vi "TDMS - File Viewer (NXG Style).vi"(8 "error in":errorcluster, 11 "file in":path) -> (0 "error out":errorcluster={"status"=TRUE, "code"=118, "source"="TDMS Open in TDMS - File Viewer with Flat Layout.vi"}, 3 "file out":path)   [LabVIEW 2020, in "NI_TDMS File Viewer.lvlib"]
doc: "Opens the .tdms file specified in the <B>file path</B> input and presents the file data in the TDMS File Viewer dialog box."
uses:
  <vilib>/Utility/TDMS File Viewer/NI_TDMS File Viewer.lvlib
  <vilib>/Utility/miscctls.llb/LVRowAndColumnTypeDef.ctl
  <vilib>/Utility/error.llb/DialogType.ctl
  <vilib>/Utility/TDMS File Viewer/Global VI for Localized Text.vi
panel:
  in  "Help":bool
  in  "File Tree":string[](tree)
  out "Property Table":string[][](table)
  in  "All":bool
  in  "Samples":i64=100000 min=-1 step=1
  in  "Start index":i64 min=0 step=1
  out "Waveform Graph":waveform(dbl)[](graph)
  in  "Value Table":i32(listbox)=-1
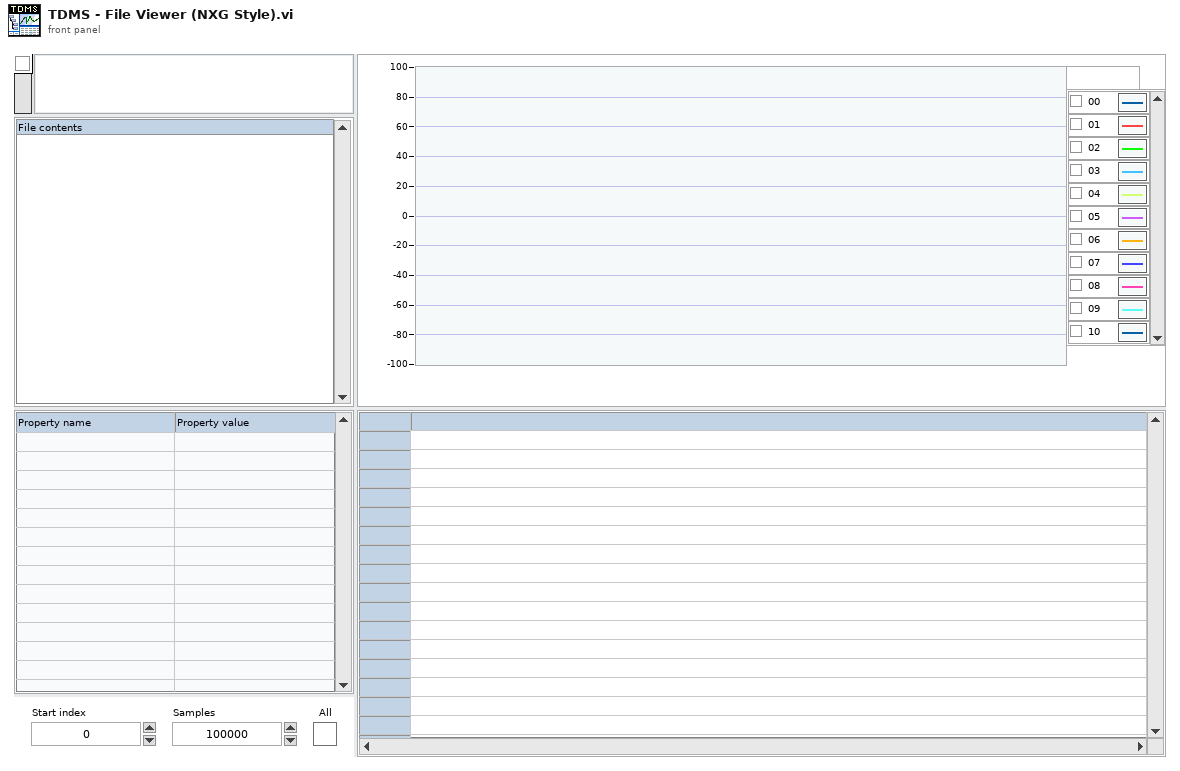
[diagram p1: front panel]
types:
  T1 = enum16{"open", "open or create", "create or replace", "create", "open (read-only)"}
  T2 = cluster{"All":bool, "Start index":i64, "Samples":i64}
  T3 = enum8{"Enabled", "Disabled", "Disabled and Grayed Out"}
  T4 = typedef "eventvkey.ctl" = enum16{"ASCII", "Enter", "Return", "Shift", "Ctrl", "Alt", "Cmd", "Opt", "Caps", "NumLock", "Clear", "Break", "Up", "Down", "Left", "Right", "Insert", "Delete", "Home", "End", "PageUp", "PageDown", "Escape", "Help", "Pause", "ScrollLock", "F1", "F2", "F3", "F4", "F5", "F6", "F7", "F8", "F9", "F10", "F11", "F12", "F13", "F14", "F15", "F16", "F17", "F18", "F19", "F20", "F21", "F22", "F23", "F24", "Play", "VolumeUp", "VolumeDown", "Mute", "Two Byte Char"}
  T5 = typedef "LVPoint32TypeDef.ctl" = cluster{"Horizontal":i32, "Vertical":i32}
  T6 = typedef "NI_TDMS File Viewer.lvlib/Table Components.ctl" = cluster{"column headers":string[], "row headers":string[], "values":string[][]}
  T7 = typedef "LVRowAndColumnTypeDef.ctl" = cluster{"Row":i32, "Column":i32}
  T8 = typedef "DialogType.ctl" = u16
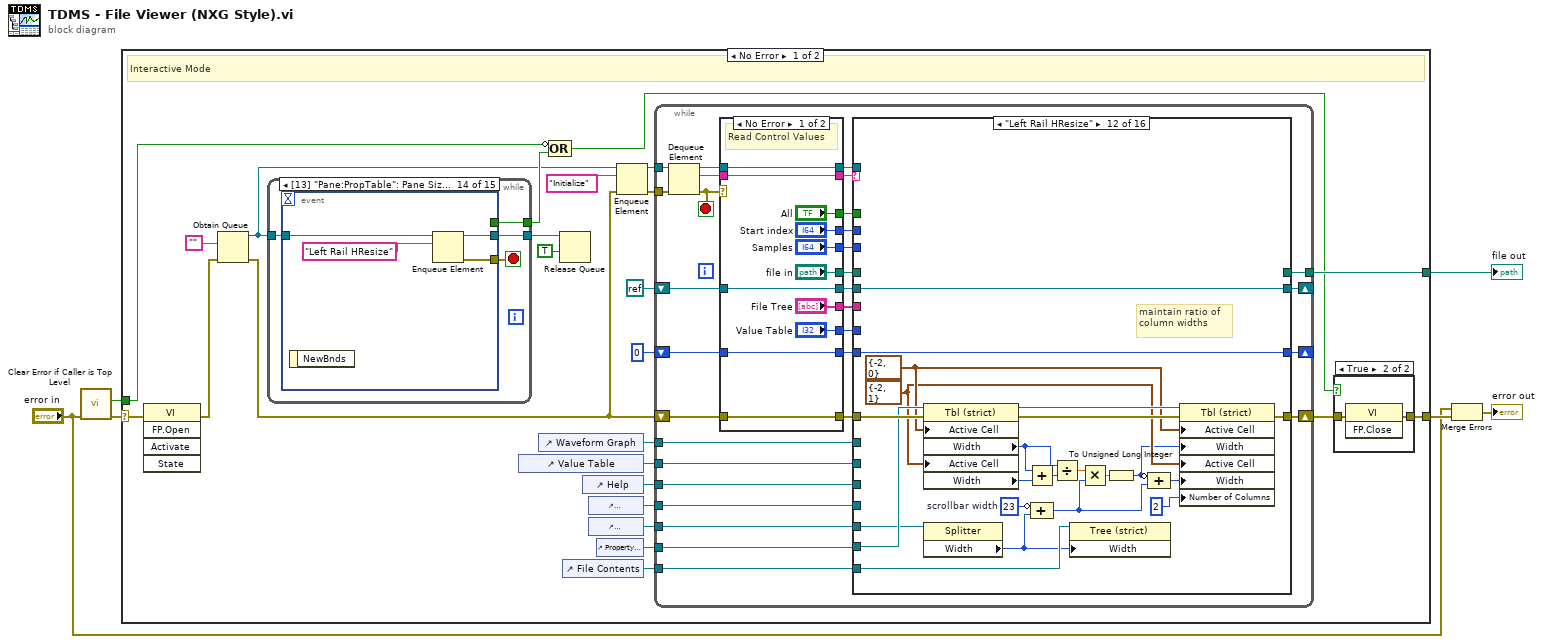
[diagram p0: block diagram]
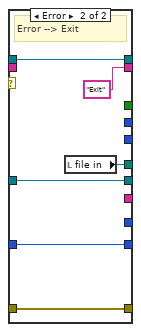
[diagram p3: hidden frame]
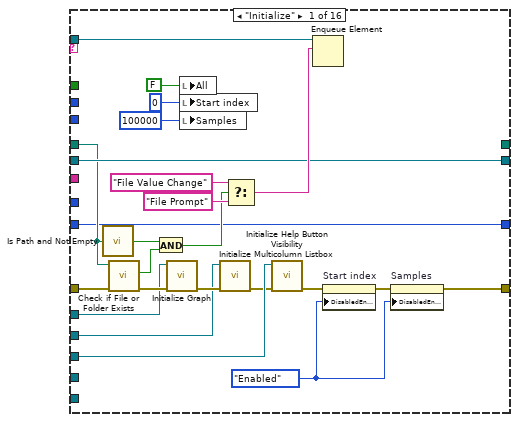
[diagram p4: hidden frame]
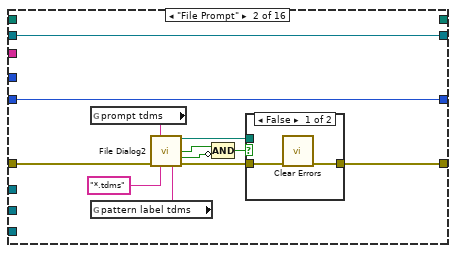
[diagram p5: hidden frame]
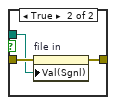
[diagram p6: hidden frame]
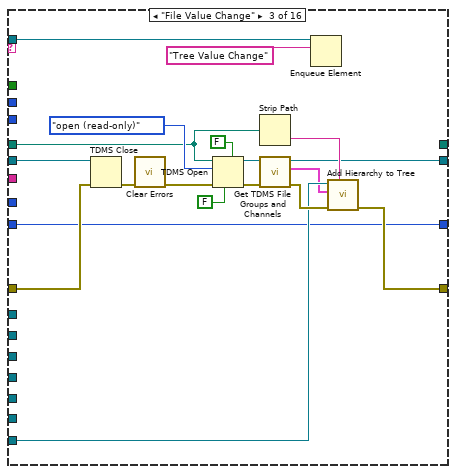
[diagram p7: hidden frame]
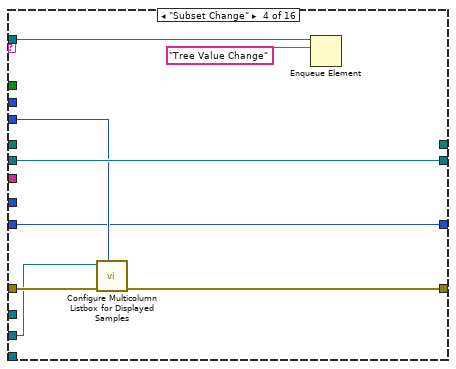
[diagram p8: hidden frame]
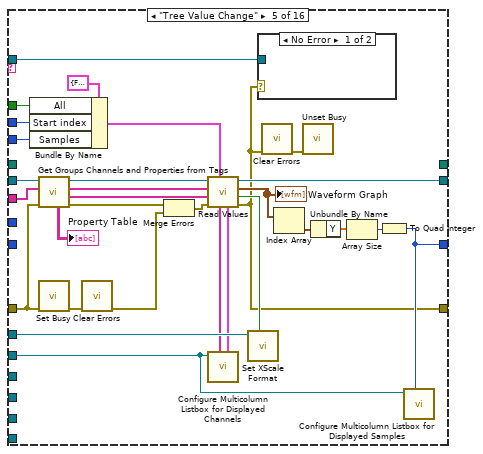
[diagram p9: hidden frame]
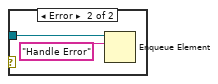
[diagram p10: hidden frame]
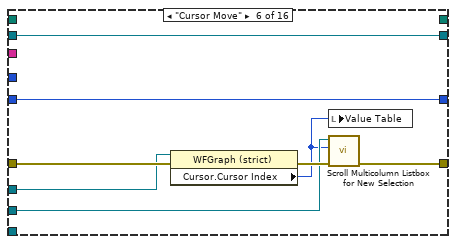
[diagram p11: hidden frame]
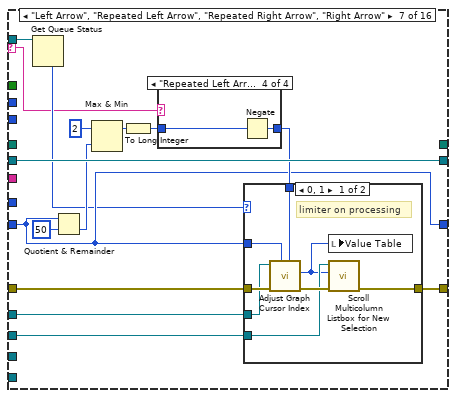
[diagram p12: hidden frame]
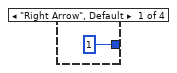
[diagram p14: hidden frame]
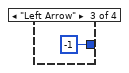
[diagram p16: hidden frame]
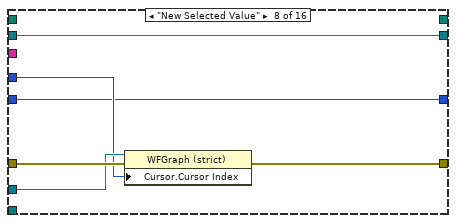
[diagram p17: hidden frame]
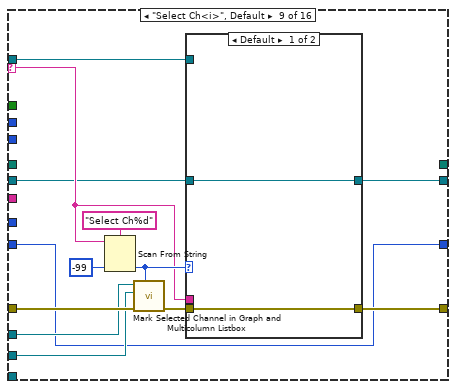
[diagram p18: hidden frame]
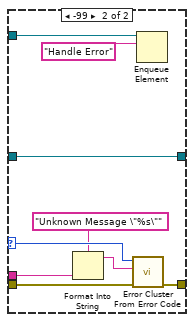
[diagram p19: hidden frame]
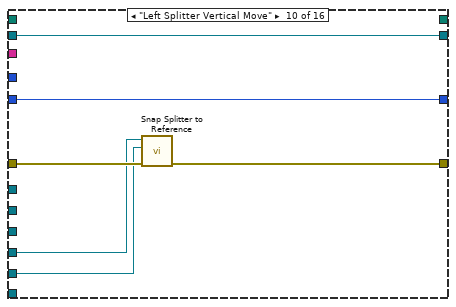
[diagram p20: hidden frame]
diagram:
  n1 = call <vilib>:"Clear Error if Caller is Top Level.vi"("error in"="error in") -> ("error out"=w6:errorcluster, "top level"=w1:bool)  [unwired: 9 in]
  n2 = case shown="No Error" w6 {
    selector: w6 -> [w11 w429]
    tunnel: [w21 _] -> w2
    tunnel: [w30 w429] -> w5
    tunnel: w1 -> [w18 _]
    frame No Error {
      # "Interactive Mode"
      n3 = invoke class="VI" method="FP.Open"(error in=w11) -> (error out=w10:errorcluster)  [unwired: 4 in, 4 out]
      n4 = Obtain Queue(element data type="", error in (no error)=w10) -> (queue out=w9:refnum<queue>, error out=w12:errorcluster)  [unwired: 3 in, 1 out]
      n5 = while {
        tunnel: [w315] -> w20
        tunnel: w9 -> [w314]
        tunnel: [w313] -> w16
        stop <- w316 stop-if-true
        n6 = event shown="[13] \"Pane:PropTable\": Pane Size" {
          selector: _ -> [_ _ _ _ _ _ _ _ _ _ _ _ _ _ _]
          dyn-events: _ -> [_ _ _ _ _ _ _ _ _ _ _ _ _ _ _]
          timeout: _ -> [_ _ _ _ _ _ _ _ _ _ _ _ _ _ _]
          tunnel: [w318 w327 w335 w350 w354 w358 w375 w392 w396 w400 w409 w413 w417 w420 w425] -> w316
          tunnel: [_ _ _ _ _ _ _ _ _ _ _ _ _ _ w427] -> w315
          tunnel: w314 -> [w319 w328 w336 w351 w355 w359 w376 w393 w397 w401 w410 w414 w418 w422 w426]
          tunnel: [w317 w326 w334 w349 w353 w357 w374 w391 w395 w399 w408 w412 w416 w421 w424] -> w313
          event "Start index", "Samples": Value Change {
            n7 = event-data() -> ()  [unwired: 1 in, 1 out]
            n8 = local read "Start index"() -> (w324:i64)
            n9 = local read "Samples"() -> (w323:i64)
            n10 = Less Than 0?(x=w323) -> (x < 0?=w322:bool)
            n11 = Equal To 0?(x=w324) -> (x = 0?=w321:bool)
            n12 = And(x=w322, y=w321) -> (x .and. y?=w320:bool)
            n13 = local write "All"(w320) -> ()
            n14 = Enqueue Element(queue=w319, element="Subset Change" ("CHM or HLP filename (lvdialog.chm)")) -> (queue out=w317:refnum<queue>, error out=w318:errorcluster)  [unwired: 2 in, 1 out]
          }
          event "All": Value Change {
            n15 = event-data() -> ("NewVal"=w330:bool)  [unwired: 1 in]
            n16 = Select(t=T3."Disabled and Grayed Out" ("Disabled"), s=w330, f=T3."Enabled" ("Disabled")) -> (s? t:f=w329:T3)
            n17 = property on="Start index" class="DigNum (strict)"("DisabledEnum"=w329) -> ()  [unwired: 2 in, 2 out]
            n18 = property on="Samples" class="DigNum (strict)"("DisabledEnum"=w329) -> ()  [unwired: 2 in, 2 out]
            n19 = Enqueue Element(queue=w328, element="Subset Change" ("CHM or HLP filename (lvdialog.chm)")) -> (queue out=w326:refnum<queue>, error out=w327:errorcluster)  [unwired: 2 in, 1 out]
          }
          event "file in": Value Change {
            n20 = event-data() -> ("OldVal"=w337:path, "NewVal"=w341:path)  [unwired: 1 in]
            n21 = call <vilib>:"Is Path and Not Empty.vi"("path"=w341) -> ("Is Path and Not Empty?"=w340:bool)  [unwired: 4 in]
            n22 = call <vilib>:"Check if File or Folder Exists.vi"("path"=w341) -> ("file or folder exists?"=w339:bool)  [unwired: 8 in, 2 out]
            n23 = And(x=w339, y=w340) -> (x .and. y?=w338:bool)
            n24 = case shown="False" w338 {
              tunnel: "File Value Change" ("CHM or HLP filename (lvdialog.chm)") -> [_ w348]
              tunnel: w337 -> [w344 _]
              tunnel: w336 -> [w343 w347]
              tunnel: [_ w346] -> w335
              tunnel: [w343 w345] -> w334
              frame False {
                n25 = local write "file in"(w344) -> ()
              }
              frame True {
                n26 = Enqueue Element(queue=w347, element=w348) -> (queue out=w345:refnum<queue>, error out=w346:errorcluster)  [unwired: 2 in, 1 out]
              }
            }
          }
          event "File Tree": Value Change {
            n27 = event-data() -> ()  [unwired: 1 in, 1 out]
            n28 = Enqueue Element(queue=w351, element="Tree Value Change" ("CHM or HLP filename (lvdialog.chm)")) -> (queue out=w349:refnum<queue>, error out=w350:errorcluster)  [unwired: 2 in, 1 out]
          }
          event "Help": Value Change {
            n29 = event-data() -> ()  [unwired: 1 in, 1 out]
            n30 = Enqueue Element(queue=w355, element="Launch Help" ("CHM or HLP filename (lvdialog.chm)")) -> (queue out=w353:refnum<queue>, error out=w354:errorcluster)  [unwired: 2 in, 1 out]
          }
          event Key Down? {
            n31 = event-data() -> ("VKey"=w362:T4)  [unwired: 1 in]
            n32 = case shown="\"Left\"" w362 {
              tunnel: [_ w367 w372] -> w360
              tunnel: TRUE ("Discard?") -> [_ w367 w372]
              tunnel: w359 -> [w363 w366 w371]
              tunnel: [_ w365 w370] -> w358
              tunnel: [w363 w364 w369] -> w357
              frame Default {
              }
              frame "Left" {
                n33 = Enqueue Element(queue=w366, element="Left Arrow" ("CHM or HLP filename (lvdialog.chm)")) -> (queue out=w364:refnum<queue>, error out=w365:errorcluster)  [unwired: 2 in, 1 out]
              }
              frame "Right" {
                n34 = Enqueue Element(queue=w371, element="Right Arrow" ("CHM or HLP filename (lvdialog.chm)")) -> (queue out=w369:refnum<queue>, error out=w370:errorcluster)  [unwired: 2 in, 1 out]
              }
            }
            n35 = event-data("Discard?"=w360) -> ()  [unwired: 1 in, 1 out]
          }
          event event type 5.0.x8000000b {
            n36 = event-data() -> ("VKey"=w379:T4)  [unwired: 1 in]
            n37 = case shown="\"Right\"" w379 {
              tunnel: [_ w384 w389] -> w378
              tunnel: TRUE ("abort (F)") -> [_ w384 w389]
              tunnel: w376 -> [w380 w383 w388]
              tunnel: [_ w382 w387] -> w375
              tunnel: [w380 w381 w386] -> w374
              frame Default {
              }
              frame "Left" {
                n38 = Enqueue Element(queue=w383, element="Repeated Left Arrow" ("CHM or HLP filename (lvdialog.chm)")) -> (queue out=w381:refnum<queue>, error out=w382:errorcluster)  [unwired: 2 in, 1 out]
              }
              frame "Right" {
                n39 = Enqueue Element(queue=w388, element="Repeated Right Arrow" ("CHM or HLP filename (lvdialog.chm)")) -> (queue out=w386:refnum<queue>, error out=w387:errorcluster)  [unwired: 2 in, 1 out]
              }
            }
            n40 = event-data("Discard?"=w378) -> ()  [unwired: 1 in, 1 out]
          }
          event "Waveform Graph": Cursor Move {
            n41 = event-data() -> ()  [unwired: 1 in, 1 out]
            n42 = Enqueue Element(queue=w393, element="Cursor Move" ("CHM or HLP filename (lvdialog.chm)")) -> (queue out=w391:refnum<queue>, error out=w392:errorcluster)  [unwired: 2 in, 1 out]
          }
          event "Value Table": Value Change {
            n43 = event-data() -> ()  [unwired: 1 in, 1 out]
            n44 = Enqueue Element(queue=w397, element="New Selected Value" ("CHM or HLP filename (lvdialog.chm)")) -> (queue out=w395:refnum<queue>, error out=w396:errorcluster)  [unwired: 2 in, 1 out]
          }
          event "Value Table": Double Click {
            n45 = event-data() -> ("CtlRef"=w407:refnum<vi>, "Coords"=w402:T5)  [unwired: 1 in]
            n46 = call <vilib>:"Coordinates to Multicolumn Listbox Column.vi"("Coords"=w402, "MulticolumnListbox in"=w407) -> ("Column"=w405:i32)  [unwired: 9 in]
            n47 = Format Into String(format string="%d", initial string="Select Ch" ("CHM or HLP filename (lvdialog.chm)"), w405) -> (resulting string=w403:string)  [unwired: 1 in, 1 out]
            n48 = Enqueue Element(queue=w401, element=w403) -> (queue out=w399:refnum<queue>, error out=w400:errorcluster)  [unwired: 2 in, 1 out]
          }
          event Mouse Leave; Mouse Up {
            n49 = event-data() -> ()  [unwired: 1 in, 1 out]
            n50 = Enqueue Element(queue=w410, element="Left Splitter Vertical Move" ("CHM or HLP filename (lvdialog.chm)")) -> (queue out=w408:refnum<queue>, error out=w409:errorcluster)  [unwired: 2 in, 1 out]
          }
          event Mouse Leave; Mouse Up {
            n51 = event-data() -> ()  [unwired: 1 in, 1 out]
            n52 = Enqueue Element(queue=w414, element="Right Splitter Vertical Move" ("CHM or HLP filename (lvdialog.chm)")) -> (queue out=w412:refnum<queue>, error out=w413:errorcluster)  [unwired: 2 in, 1 out]
          }
          event Pane Size {
            n53 = event-data() -> ()  [unwired: 1 in, 1 out]
            n54 = Enqueue Element(queue=w418, element="Graph Resize" ("CHM or HLP filename (lvdialog.chm)")) -> (queue out=w416:refnum<queue>, error out=w417:errorcluster)  [unwired: 2 in, 1 out]
          }
          event Pane Size {
            n55 = event-data() -> ()  [unwired: 1 in, 1 out]
            n56 = Enqueue Element(queue=w422, element="Left Rail HResize" ("CHM or HLP filename (lvdialog.chm)")) -> (queue out=w421:refnum<queue>, error out=w420:errorcluster)  [unwired: 2 in, 1 out]
          }
          event Panel Close? {
            w425 = errorcluster {"status"=TRUE, "code"=0, "source"=""}  # Stop
            w427 = TRUE ("Discard?")
            n57 = event-data() -> ()  [unwired: 1 in, 1 out]
            n58 = Enqueue Element(queue=w426, element="Exit" ("CHM or HLP filename (lvdialog.chm)")) -> (queue out=w424:refnum<queue>)  [unwired: 2 in, 2 out]
            n59 = event-data("Discard?"=w427) -> ()  [unwired: 1 in, 1 out]
          }
        }
      }
      n60 = control-ref of="Value Table"() -> (w28:refnum<vi>)
      n61 = control-ref of="Waveform Graph"() -> (w24:refnum<vi>)
      n62 = Compound Arithmetic op=OR(invert w18, w20) -> (w7:bool)
      n63 = Release Queue(queue=w16, force destroy? (F)=TRUE) -> ()  [unwired: 1 in, 3 out]
      n64 = control-ref of="File Contents"() -> (w27:refnum<vi>)
      n65 = control-ref of="Help"() -> (w26:refnum<vi>)
      n66 = control-ref of="Splitter:ValueTableTop"() -> (w23:refnum<vi>)
      n67 = control-ref of="Splitter:PropTableTop"() -> (w22:refnum<vi>)
      n68 = control-ref of="Property Table"() -> (w8:refnum<vi>)
      n69 = Enqueue Element(queue=w9, element="Initialize" ("CHM or HLP filename (lvdialog.chm)"), error in (no error)=w12) -> (queue out=w17:refnum<queue>, error out=w14:errorcluster)  [unwired: 1 in, 1 out]
      n70 = while {
        tunnel: w17 -> [w61]
        shift-right: [w50] -> _
        shift-left: refnum<k0> refnum -> [w51]
        shift-right: [w62] -> w31
        shift-left: w12 -> [w63]
        tunnel: w28 -> [w49]
        tunnel: w27 -> [w48]
        tunnel: w26 -> [w47]
        tunnel: w24 -> [w45]
        tunnel: w23 -> [w44]
        tunnel: w22 -> [w43]
        tunnel: [w42] -> w21
        shift-right: [w39] -> _
        shift-left: i64 0 -> [w40]
        tunnel: w14 -> [w36]
        tunnel: w8 -> [w35]
        stop <- w60 stop-if-true
        n71 = Dequeue Element(queue=w61, error in (no error)=w36) -> (queue out=w38:refnum<queue>, element=w58:string, error out=w60:errorcluster)  [unwired: 1 in, 1 out]
        n72 = case shown="No Error" w60 {
          tunnel: [w74 "Exit" ("element")] -> w59
          tunnel: w58 -> [w74 _]
          tunnel: ["file in" w78] -> w57
          tunnel: ["File Tree" _] -> w56
          tunnel: ["Samples" _] -> w55
          tunnel: ["Start index" _] -> w54
          tunnel: ["All" _] -> w53
          tunnel: [w68 w79] -> w52
          tunnel: w51 -> [w68 w79]
          tunnel: [w75 w81] -> w64
          tunnel: w63 -> [w75 w81]
          tunnel: ["Value Table" _] -> w46
          tunnel: [w66 w77] -> w41
          tunnel: w40 -> [w66 w77]
          tunnel: [w65 w76] -> w37
          tunnel: w38 -> [w65 w76]
          frame No Error {
            # "Read Control Values"
          }
          frame Error {
            # "Error --> Exit"
            n73 = local read "file in"() -> (w78:path)
          }
        }
        n74 = case shown="\"Left Rail HResize\"" w59 {
          selector: w59 -> [_ _ _ _ _ _ w190 _ w228 _ _ _ _ _ _ _]
          tunnel: w57 -> [w98 _ w124 _ _ _ _ _ _ _ _ _ _ _ w303 _]
          tunnel: w56 -> [_ _ _ _ w158 _ _ _ _ _ _ _ _ _ _ _]
          tunnel: w55 -> [_ _ _ w144 w171 _ _ _ _ _ _ _ _ _ _ _]
          tunnel: w54 -> [_ _ _ _ w172 _ _ _ _ _ _ _ _ _ _ _]
          tunnel: w53 -> [_ _ _ _ w173 _ _ _ _ _ _ _ _ _ _ _]
          tunnel: w49 -> [w85 _ _ w145 w161 w184 w200 _ w231 _ _ _ _ _ _ _]
          tunnel: w52 -> [w99 w109 w130 w147 w175 w186 w202 w222 w225 w252 w258 w282 w287 w292 w305 w308]
          tunnel: [w99 w109 w126 w147 w174 w186 w202 w222 w226 w252 w258 w282 w287 w292 refnum<k0> refnum w308] -> w50
          tunnel: w64 -> [w105 w117 w140 w149 w156 w189 w204 w223 w237 w254 w259 w280 w290 w294 w306 w311]
          tunnel: w48 -> [_ _ w129 _ _ _ _ _ _ _ _ w262 _ _ _ _]
          tunnel: [w102 w115 w136 w148 w157 w187 w203 w224 w235 w253 w260 w277 w288 w293 w306 w312] -> w62
          tunnel: w47 -> [w101 _ _ _ _ _ _ _ _ _ _ _ _ _ _ _]
          tunnel: w46 -> [_ _ _ _ _ _ _ w220 _ _ _ _ _ _ _ _]
          tunnel: w45 -> [w97 _ _ _ w169 w185 w201 w221 w232 _ _ _ w286 _ _ _]
          tunnel: w44 -> [_ _ _ _ _ _ _ _ _ w251 w257 _ w285 _ _ _]
          tunnel: w43 -> [_ _ _ _ _ _ _ _ _ w250 w256 w273 w284 _ _ _]
          tunnel: [_ _ _ _ _ _ _ _ _ _ _ _ _ _ w303 _] -> w42
          tunnel: w41 -> [w87 w106 w125 w143 _ w182 w198 w219 w229 w249 w255 w281 w283 w291 w302 w307]
          tunnel: [w87 w106 w125 w143 w160 w182 w198 w219 w229 w249 w255 w281 w283 w291 w302 w307] -> w39
          tunnel: w37 -> [w82 _ w123 w142 w150 _ w192 _ w227 _ _ _ _ _ _ _]
          tunnel: w35 -> [_ _ _ _ _ _ _ _ _ _ _ w279 _ _ _ _]
          frame "Initialize" {
            w88 = T3."Enabled" ("Disabled")
            n75 = call <vilib>:"Is Path and Not Empty.vi"("path"=w98) -> ("Is Path and Not Empty?"=w94:bool)  [unwired: 4 in]
            n76 = call <vilib>:"Check if File or Folder Exists.vi"("error in (no error)"=w105, "path"=w98) -> ("error out"=w104:errorcluster, "file or folder exists?"=w93:bool)  [unwired: 7 in, 1 out]
            n77 = And(x=w94, y=w93) -> (x .and. y?=w92:bool)
            n78 = call <vilib>:"Initialize Graph.vi"("error in"=w104, "WaveformGraph"=w97) -> ("error out"=w86:errorcluster)  [unwired: 9 in]
            n79 = local write "All"(FALSE ("All")) -> ()
            n80 = local write "Start index"(i64 0 ("Start index")) -> ()
            n81 = local write "Samples"(i64 100000 ("Samples")) -> ()
            n82 = call <vilib>:"Initialize Multicolumn Listbox.vi"("error in"=w86, "MulticolumnListbox"=w85) -> ("error out"=w84:errorcluster)  [unwired: 9 in]
            n83 = Select(t="File Value Change" ("CHM or HLP filename (lvdialog.chm)"), s=w92, f="File Prompt" ("CHM or HLP filename (lvdialog.chm)")) -> (s? t:f=w100:string)
            n84 = call <vilib>:"Initialize Help Button Visibility.vi"("error in"=w84, "Help"=w101) -> ("error out"=w83:errorcluster)  [unwired: 9 in]
            n85 = Enqueue Element(queue=w82, element=w100) -> ()  [unwired: 2 in, 3 out]
            n86 = property on="Start index" class="DigNum (strict)"(error in=w83, "DisabledEnum"=w88) -> (error out=w103:errorcluster)  [unwired: 1 in, 1 out]
            n87 = property on="Samples" class="DigNum (strict)"(error in=w103, "DisabledEnum"=w88) -> (error out=w102:errorcluster)  [unwired: 1 in, 1 out]
          }
          frame "File Prompt" {
            n88 = global read "Global VI for Localized Text.vi" "prompt tdms"() -> (w113:string)
            n89 = global read "Global VI for Localized Text.vi" "pattern label tdms"() -> (w112:string)
            n90 = call "File Dialog2"("prompt"=w113, "error in"=w117, "pattern (all files)"="*.tdms", "pattern label"=w112) -> ("selected path"=w110:path, "exists"=w108:bool, "cancelled"=w107:bool, "error out"=w116:errorcluster)  [unwired: 3 in, 5 out]
            n91 = Compound Arithmetic op=AND(w108, invert w107) -> (w111:bool)
            n92 = case shown="False" w111 {
              tunnel: w116 -> [w119 w122]
              tunnel: [w118 w121] -> w115
              tunnel: w110 -> [_ w120]
              frame False {
                n93 = call <vilib>:"Clear Errors.vi"("error in (no error)"=w119) -> ("error out"=w118:errorcluster)  [unwired: 5 in, 1 out]
              }
              frame True {
                n94 = property on="file in" class="Path"(error in=w122, "Val(Sgnl)"=w120) -> (error out=w121:errorcluster)  [unwired: 1 in, 1 out]
              }
            }
          }
          frame "File Value Change" {
            n95 = TDMS Close(8:w140, 11:w130) -> (0:w139:errorcluster)  [unwired: 1 out]
            n96 = call <vilib>:"Clear Errors.vi"("error in (no error)"=w139) -> ("error out"=w138:errorcluster)  [unwired: 5 in, 1 out]
            n97 = TDMS Open(5:FALSE ("create index file? (T)"), 6:FALSE ("disable buffering (T)"), 8:w138, 10:T1."open (read-only)" ("operation"), 11:w124) -> (0:w141:errorcluster, 3:w131:refnum<k34>)  [unwired: 2 in]
            n98 = Strip Path(path=w124) -> (name=w128:string)  [unwired: 1 out]
            n99 = call <vilib>:"Get TDMS File Groups and Channels.vi"("error in"=w141, "TDMS ref in"=w131) -> ("error out"=w137:errorcluster, "file contents"=w127:cluster{string, string[]}[], "TDMS ref out"=w126:refnum<k34>)  [unwired: 7 in]
            n100 = Enqueue Element(queue=w123, element="Tree Value Change" ("CHM or HLP filename (lvdialog.chm)")) -> ()  [unwired: 2 in, 3 out]
            n101 = call <vilib>:"Add Hierarchy to Tree.vi"("file name"=w128, "error in"=w137, "file contents"=w127, "file tree refnum"=w129) -> ("error out"=w136:errorcluster)  [unwired: 7 in]
          }
          frame "Subset Change" {
            n102 = call <vilib>:"Configure Multicolumn Listbox for Displayed Samples.vi"("Samples"=w144, "error in"=w149, "MulticolumnListbox in"=w145) -> ("error out"=w148:errorcluster)  [unwired: 7 in, 1 out]
            n103 = Enqueue Element(queue=w142, element="Tree Value Change") -> ()  [unwired: 2 in, 3 out]
          }
          frame "Tree Value Change" {
            n104 = Bundle By Name(cluster=T2 {"All"=FALSE, "Start index"=0, "Samples"=0}, "All"=w173, "Start index"=w172, "Samples"=w171) -> (w170:T2)
            n105 = call <vilib>:"Get Groups Channels and Properties from Tags.vi"("error in"=w156, "File Tree"=w158, "tdms file in"=w175) -> ("error out"=w153:errorcluster, "channel names out"=w178:string[], "group names out"=w177:string[], "tdms file out"=w176:refnum<k34>, "property table"=→"Property Table":string[][])  [unwired: 2 in]
            n106 = call <vilib>:"Set Busy.vi"("error in (no error)"=w156) -> ("error out"=w159:errorcluster)  [unwired: 9 in, 1 out]
            n107 = call <vilib>:"Clear Errors.vi"("error in (no error)"=w159) -> ("error out"=w155:errorcluster)  [unwired: 5 in, 1 out]
            n108 = Merge Errors(w153, w155) -> (w154:errorcluster)
            n109 = call <vilib>:"Read Values.vi"("read subset"=w170, "error in"=w154, "channel names"=w178, "group names"=w177, "tdms file"=w176) -> ("error out"=w157:errorcluster, "waveform timestamps = 0"=w164:bool, "waveform values"=w165:waveform(dbl)[], "tdms file out"=w174:refnum<k34>, "table values"=w168:T6, "widest value strings"=w166:string[])  [unwired: 1 in]
            "Waveform Graph" <- w165
            n110 = call <vilib>:"Configure Multicolumn Listbox for Displayed Channels.vi"("table values"=w168, "widest value strings"=w166, "MulticolumnListbox in"=w161) -> ()  [unwired: 7 in]
            n111 = call <vilib>:"Set XScale Format.vi"("timestamp eq 0"=w164, "Waveform Graph"=w169) -> ()  [unwired: 8 in]
            n112 = case shown="No Error" w157 {
              tunnel: w150 -> [_ w180]
              frame No Error {
              }
              frame Error {
                n113 = Enqueue Element(queue=w180, element="Handle Error") -> ()  [unwired: 2 in, 3 out]
              }
            }
            n114 = call <vilib>:"Clear Errors.vi"("error in (no error)"=w157) -> ("error out"=w179:errorcluster)  [unwired: 5 in, 1 out]
            n115 = Index Array(array=w165) -> (element=w162:waveform(dbl))  [unwired: 1 in]
            n116 = call <vilib>:"Unset Busy.vi"("error in (no error)"=w179) -> ()  [unwired: 10 in, 1 out]
            n117 = Unbundle By Name(w162) -> ("Y"=w163:dbl[])
            n118 = Array Size(array=w163) -> (size(s)=w152:i32)
            n119 = To Quad Integer(1:w152) -> (0:w160:i64)
            n120 = call <vilib>:"Configure Multicolumn Listbox for Displayed Samples.vi"("Samples"=w160, "MulticolumnListbox in"=w161) -> ()  [unwired: 8 in, 2 out]
          }
          frame "Cursor Move" {
            n121 = property class="WFGraph (strict)"(reference=w185, error in=w189) -> (error out=w188:errorcluster, "Cursor.Cursor Index"=w183:i32)  [unwired: 1 out]
            n122 = local write "Value Table"(w183) -> ()
            n123 = call <vilib>:"Scroll Multicolumn Listbox for New Selection.vi"("error in"=w188, "new index"=w183, "MulticolumnListbox"=w184) -> ("error out"=w187:errorcluster)  [unwired: 8 in]
          }
          frame "Left Arrow", "Repeated Left Arrow", "Repeated Right Arrow", "Right Arrow" {
            n124 = Get Queue Status(queue=w192) -> (# elements in queue=w191:i32)  [unwired: 2 in, 7 out]
            n125 = Quotient & Remainder(x=w198, y=i64 50) -> (floor(x/y)=w196:i64)  [unwired: 1 out]
            n126 = Max & Min(x=i64 2, y=w196) -> (max(x,y)=w194:i64)  [unwired: 1 out]
            n127 = To Long Integer(number=w194) -> (32bit integer=w193:i32)
            n128 = case shown="\"Repeated Left Arrow\"" w190 {
              tunnel: [1 w215 -1 w217] -> w199
              tunnel: w193 -> [_ w215 _ w218]
              frame "Right Arrow", Default {
              }
              frame "Repeated Right Arrow" {
              }
              frame "Left Arrow" {
              }
              frame "Repeated Left Arrow" {
                n129 = Negate(x=w218) -> (-x=w217:i32)
              }
            }
            n130 = case shown="0, 1" w191 {
              tunnel: w201 -> [w209 _]
              tunnel: w204 -> [w212 w213]
              tunnel: w200 -> [w208 _]
              tunnel: [w210 w213] -> w203
              tunnel: w199 -> [w206 _]
              tunnel: w198 -> [w205 _]
              frame 0, 1 {
                # "limiter on processing"
                n131 = call <vilib>:"Adjust Graph Cursor Index.vi"("index adjustment"=w206, "Plot 0 samples"=w205, "error in"=w212, "WaveformGraph in"=w209) -> ("error out"=w211:errorcluster, "adjusted index"=w207:i32)  [unwired: 6 in]
                n132 = local write "Value Table"(w207) -> ()
                n133 = call <vilib>:"Scroll Multicolumn Listbox for New Selection.vi"("error in"=w211, "new index"=w207, "MulticolumnListbox"=w208) -> ("error out"=w210:errorcluster)  [unwired: 8 in]
              }
              frame Default {
                # "When message backlog is high, we don't execute time consuming code to adjust graph cursor position and value table"
              }
            }
          }
          frame "New Selected Value" {
            n134 = property class="WFGraph (strict)"(reference=w221, error in=w223, "Cursor.Cursor Index"=w220) -> (error out=w224:errorcluster)  [unwired: 1 out]
          }
          frame "Select Ch<i>", Default {
            n135 = Scan From String(format string="Select Ch%d", input string=w228, default 1=-99 ("default value 1")) -> (output 1=w230:i32)  [unwired: 2 in, 3 out]
            n136 = call <vilib>:"Mark Selected Channel in Graph and Multicolumn Listbox.vi"("selected channel"=w230, "error in"=w237, "Value Table"=w231, "WaveformGraph"=w232) -> ("error out"=w236:errorcluster)  [unwired: 7 in]
            n137 = case shown="Default" w230 {
              selector: w230 -> [_ w246]
              tunnel: w236 -> [w239 w248]
              tunnel: [w239 w247] -> w235
              tunnel: w228 -> [_ w244]
              tunnel: w227 -> [_ w241]
              tunnel: [w238 w240] -> w226
              tunnel: w225 -> [w238 w240]
              frame Default {
              }
              frame -99 {
                n138 = Format Into String(format string="Unknown Message \"%s\"", w244) -> (resulting string=w243:string)  [unwired: 2 in, 1 out]
                n139 = call <vilib>:"Error Cluster From Error Code.vi"("error in (no error)"=w248, "error message (\"\")"=w243, "error code (0)"=w246) -> ("error out"=w247:errorcluster)  [unwired: 6 in]
                n140 = Enqueue Element(queue=w241, element="Handle Error") -> ()  [unwired: 2 in, 3 out]
              }
            }
          }
          frame "Left Splitter Vertical Move" {
            n141 = call <vilib>:"Snap Splitter to Reference.vi"("error in"=w254, "splitter on move"=w250, "reference splitter"=w251) -> ("error out"=w253:errorcluster)  [unwired: 8 in]
          }
          frame "Right Splitter Vertical Move" {
            n142 = call <vilib>:"Snap Splitter to Reference.vi"("error in"=w259, "splitter on move"=w257, "reference splitter"=w256) -> ("error out"=w260:errorcluster)  [unwired: 8 in]
          }
          frame "Left Rail HResize" {
            w263 = u32 23  # scrollbar width
            w274 = T7 {"Row"=-2, "Column"=1} ("Active Cell:Active Cell")
            w275 = T7 {"Row"=-2, "Column"=0} ("Active Cell:Active Cell")
            # "maintain ratio of column widths"
            n143 = property class="Tbl (strict)"(reference=w279, error in=w280, "Active Cell"=w275, "Active Cell"=w274) -> (reference out=w276:refnum<vi>, error out=w278:errorcluster, "Width"=w270:u32, "Width"=w272:u32)
            n144 = property class="Splitter"(reference=w273) -> ("Width"=w261:u32)  [unwired: 1 in, 2 out]
            n145 = Add(x=w270, y=w272) -> (x+y=w271:u32)
            n146 = Compound Arithmetic op=ADD(invert w263, w261) -> (w264:u32)
            n147 = Divide(x=w270, y=w271) -> (x/y=w269:dbl)
            n148 = property class="Tree (strict)"(reference=w262, "Width"=w261) -> ()  [unwired: 1 in, 2 out]
            n149 = Multiply(x=w269, y=w264) -> (x*y=w268:dbl)
            n150 = To Unsigned Long Integer(number=w268) -> (unsigned 32bit integer=w267:u32)
            n151 = Compound Arithmetic op=ADD(invert w267, w264) -> (w266:u32)
            n152 = property class="Tbl (strict)"(reference=w276, error in=w278, "Active Cell"=w275, "Width"=w267, "Active Cell"=w274, "Width"=w266, "Number of Columns"=u32 2) -> (error out=w277:errorcluster)  [unwired: 1 out]
          }
          frame "Graph Resize" {
            n153 = call <vilib>:"Set Waveform Graph LegNumRows.vi"("error in"=w290, "WaveformGraph"=w286) -> ("error out"=w289:errorcluster)  [unwired: 9 in]
            n154 = call <vilib>:"Snap Splitter to Reference.vi"("error in"=w289, "splitter on move"=w284, "reference splitter"=w285) -> ("error out"=w288:errorcluster)  [unwired: 8 in]
          }
          frame "Handle Error" {
            n155 = case shown="Error .." w294 {
              selector: w294 -> [w295 w300]
              tunnel: [w295 w299] -> w293
              frame No Error {
                # "No Trouble Found"
              }
              frame Error {
                w298 = T8 4 items=["no dialog", "OK message", "continue or stop message", "OK message + warnings", "continue/stop + warnings"] ("type of dialog (OK msg:1)")
                # "Report errors"
                n156 = Unbundle By Name(w300) -> ("code"=w297:i32, "source"=w296:string)
                n157 = call <vilib>:"Simple Error Handler.vi"("error code (no error:0)"=w297, "error source (\" \")"=w296, "type of dialog (OK msg:1)"=w298, "error in (no error)"=w300) -> ("error out"=w301:errorcluster)  [unwired: 1 in, 4 out]
                n158 = call <vilib>:"Clear Errors.vi"("error in (no error)"=w301) -> ("error out"=w299:errorcluster)  [unwired: 5 in, 1 out]
              }
            }
          }
          frame "", "Exit" {
            n159 = TDMS Close(8:w306, 11:w305) -> ()  [unwired: 2 out]
          }
          frame "Launch Help" {
            n160 = call <vilib>:"Launch Help.vi"("error in"=w311, "CHM or HLP filename (lvdialog.chm)"="lvdialog.chm", "HTML filename"="tdms_file_viewer_db.html") -> ("error out"=w312:errorcluster)  [unwired: 4 out]
          }
        }
      }
      n161 = case shown="True" w7 {
        tunnel: w31 -> [w32 w34]
        tunnel: [w32 w33] -> w30
        frame False {
        }
        frame True {
          n162 = invoke class="VI" method="FP.Close"(error in=w34) -> (error out=w33:errorcluster)  [unwired: 2 in, 2 out]
        }
      }
    }
    frame Error {
      # "If TDMS File Viewer running as subVI, input error immediately returns."
    }
  }
  "file out" <- w2
  n163 = Merge Errors("error in", w5) -> (→"error out":errorcluster)
